vi "Close.vi"(8 "error in (no error)":errorcluster, 11 "Dynamixel Motor in":refnum<class "Dynamixel Motor.lvclass">) -> (0 "error out":errorcluster)   [LabVIEW 2016, in "Dynamixel Motor.lvclass"]
doc: "Performs an instrument error query before terminating the software connection to the instrument."
uses:
  <instrlib>/Dynamixel Motor/HAIOL/Dynamixel Motor.lvclass
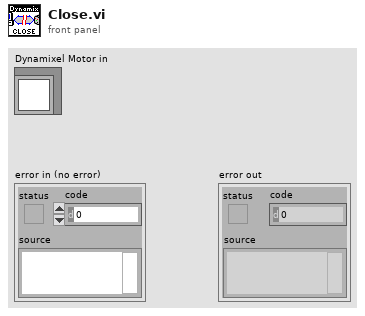
[diagram p1: front panel]
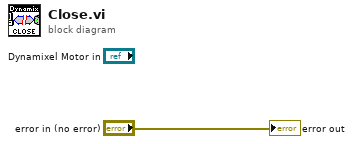
[diagram p0: block diagram]
diagram:
  "error out" <- "error in (no error)"
